vi "Ramping direction.vi"(2 "At target":bool, 3 "Actual targget [T]":dbl format="%#_13g", 4 "Actual output [T]":dbl format="%#_13g") -> (1 "Ramping direction":T1)   [LabVIEW 2022 SP3, in "Magnet module.lvlib"]
uses:
  Magnet module.lvlib
  ctl/RampingOutput.ctl
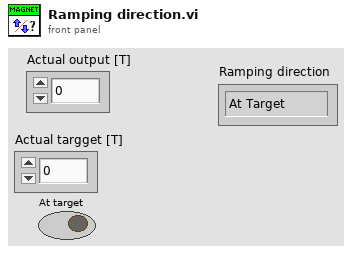
[diagram p1: front panel]
types:
  T1 = typedef "Magnet module.lvlib/RampingOutput.ctl" = enum16{"At Target", "Go up", "Go down"}
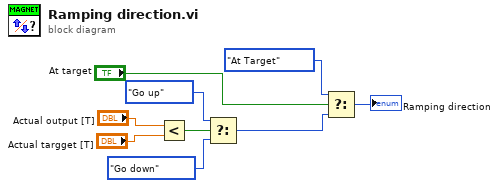
[diagram p0: block diagram]
diagram:
  n1 = Less?(x="Actual output [T]", y="Actual targget [T]") -> (x < y?=w5:bool)
  n2 = Select(t=RampingOutput."Go up" ("Ramping output"), s=w5, f=RampingOutput."Go down") -> (s? t:f=w1:T1)
  n3 = Select(t=RampingOutput."At Target" ("f"), s="At target", f=w1) -> (s? t:f=→"Ramping direction":T1)
